vi "CalcDir.vi"(9 "DirectionY":i8, 10 "DirectionX":i8, 11 "Direction in":T1) -> (3 "Direction out":T1)   [LabVIEW 2019, in "RT_Game.lvlib" / "SnakeGame.lvclass"]
uses:
  SnakeGame.lvclass
  Direction.ctl
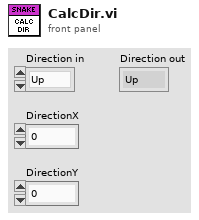
[diagram p1: front panel]
types:
  T1 = typedef "RT_Game.lvlib/SnakeGame.lvclass/Direction.ctl" = enum16{"Up", "Left", "Down", "Right"}
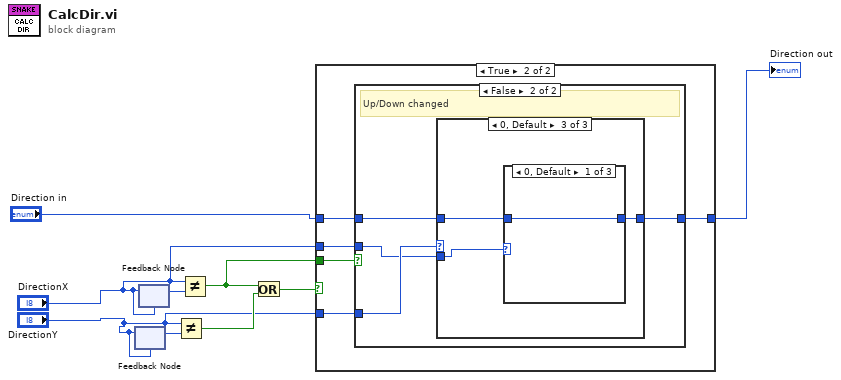
[diagram p0: block diagram]
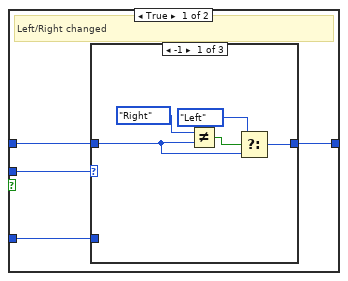
[diagram p3: hidden frame]
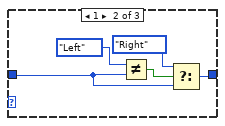
[diagram p4: hidden frame]
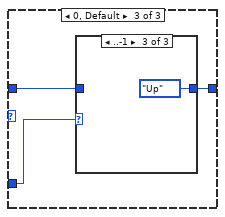
[diagram p5: hidden frame]
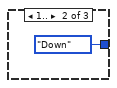
[diagram p7: hidden frame]
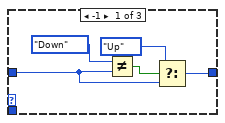
[diagram p8: hidden frame]
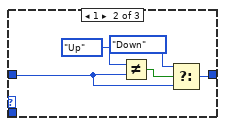
[diagram p9: hidden frame]
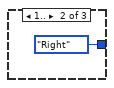
[diagram p10: hidden frame]
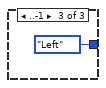
[diagram p11: hidden frame]
diagram:
  n1 = feedback #1("DirectionY") -> (w2:i8)
  n2 = feedback-in #1("DirectionY") -> ()
  n3 = feedback #2("DirectionX") -> (w1:i8)
  n4 = feedback-in #2("DirectionX") -> ()
  n5 = Not Equal?(x="DirectionY", y=w2) -> (x != y?=w5:bool)
  n6 = Not Equal?(x="DirectionX", y=w1) -> (x != y?=w7:bool)
  n7 = Or(x=w7, y=w5) -> (x .or. y?=w6:bool)
  n8 = case shown="True" w6 {
    tunnel: "DirectionX" -> [_ w14]
    tunnel: "DirectionY" -> [_ w11]
    tunnel: w7 -> [_ w15]
    tunnel: "Direction in" -> [w10 w13]
    tunnel: [w10 w12] -> w8
    frame False {
    }
    frame True {
      n9 = case shown="False" w15 {
        tunnel: w14 -> [w19 w36]
        tunnel: w13 -> [w18 w39]
        tunnel: [w17 w38] -> w12
        tunnel: w11 -> [w16 w37]
        frame True {
          # "Left/Right changed"
          n10 = case shown="-1" w19 {
            tunnel: [w22 w25 w31] -> w17
            tunnel: w18 -> [w23 w26 w30]
            tunnel: w16 -> [_ _ w32]
            frame -1 {
              n11 = Not Equal?(x=Direction."Right", y=w23) -> (x != y?=w21:bool)
              n12 = Select(t=Direction."Left", s=w21, f=w23) -> (s? t:f=w22:T1)
            }
            frame 1 {
              n13 = Not Equal?(x=Direction."Left", y=w26) -> (x != y?=w29:bool)
              n14 = Select(t=Direction."Right", s=w29, f=w26) -> (s? t:f=w25:T1)
            }
            frame 0, Default {
              n15 = case shown="..-1" w32 {
                tunnel: [w33 Direction."Down" ("Direction") Direction."Up" ("Direction")] -> w31
                tunnel: w30 -> [w33 _ _]
                frame 0, Default {
                }
                frame 1.. {
                }
                frame ..-1 {
                }
              }
            }
          }
        }
        frame False {
          # "Up/Down changed"
          n16 = case shown="0, Default" w37 {
            tunnel: [w42 w45 w51] -> w38
            tunnel: w39 -> [w43 w46 w50]
            tunnel: w36 -> [_ _ w52]
            frame -1 {
              n17 = Not Equal?(x=Direction."Down", y=w43) -> (x != y?=w41:bool)
              n18 = Select(t=Direction."Up", s=w41, f=w43) -> (s? t:f=w42:T1)
            }
            frame 1 {
              n19 = Not Equal?(x=Direction."Up", y=w46) -> (x != y?=w49:bool)
              n20 = Select(t=Direction."Down", s=w49, f=w46) -> (s? t:f=w45:T1)
            }
            frame 0, Default {
              n21 = case shown="0, Default" w52 {
                tunnel: [w53 Direction."Right" ("Direction") Direction."Left" ("Direction")] -> w51
                tunnel: w50 -> [w53 _ _]
                frame 0, Default {
                }
                frame 1.. {
                }
                frame ..-1 {
                }
              }
            }
          }
        }
      }
    }
  }
  "Direction out" <- w8
